vi "MOVIE_setup_acquisition_sCMOS.vi"(5 "Exposure time":dbl, 6 "Movie number":i32, 7 "Handle in":u32, 8 "error in":errorcluster, 9 "Movie folder name":string, 10 "Acquiring":bool, 11 "frames":i32) -> (0 "error out":errorcluster, 3 "t0":dbl)   [LabVIEW 2015]
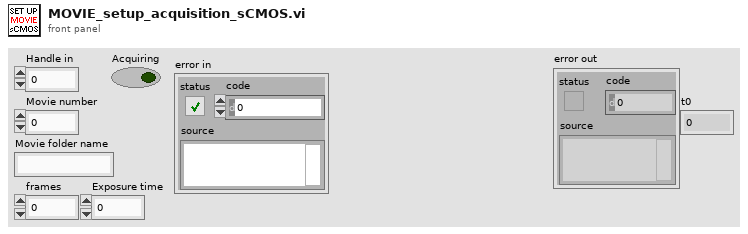
[diagram p1: front panel]
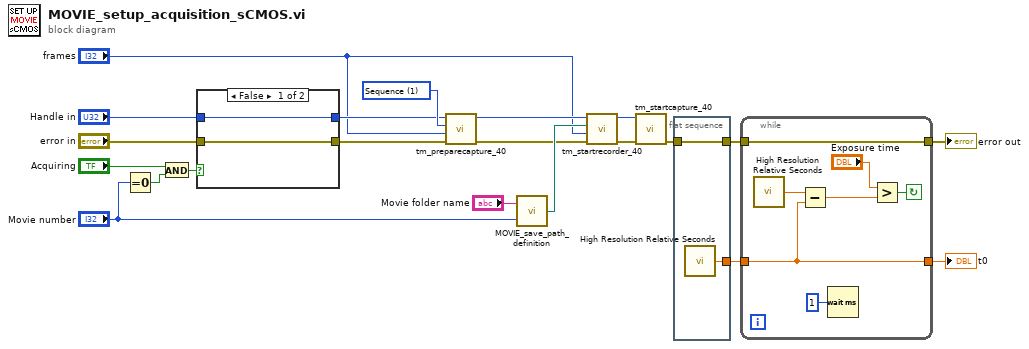
[diagram p0: block diagram]
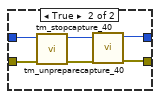
[diagram p2: hidden frame]
diagram:
  w19 = 1 items=["Snap", "Sequence"] ("Capture mode")
  n1 = Equal To 0?(x="Movie number") -> (x = 0?=w4:bool)
  n2 = And(x="Acquiring", y=w4) -> (x .and. y?=w2:bool)
  n3 = case shown="False" w2 {
    tunnel: [w23 w25] -> w14
    tunnel: "error in" -> [w23 w29]
    tunnel: "Handle in" -> [w22 w28]
    tunnel: [w22 w24] -> w15
    frame False {
    }
    frame True {
      n4 = call <userlib>:"tm_stopcapture_40.vi"("error in (no error)"=w29, "Handle in"=w28) -> ("error out"=w27:errorcluster, "Handle out"=w26:u32)  [unwired: 8 in]
      n5 = call <userlib>:"tm_unpreparecapture_40.vi"("error in (no error)"=w27, "Handle in"=w26) -> ("error out"=w25:errorcluster, "Handle out"=w24:u32)  [unwired: 8 in]
    }
  }
  n6 = call <userlib>:"tm_preparecapture_40.vi"("error in (no error)"=w14, "Frames"="frames", "Capture mode"=w19, "Handle in"=w15) -> ("error out"=w11:errorcluster, "Handle out"=w18:u32)  [unwired: 4 in, 2 out]
  n7 = call "MOVIE_save_path_definition.vi"("Movie number"="Movie number", "Movie folder name"="Movie folder name") -> ("Movie path"=w17:path)
  n8 = call <userlib>:"tm_startrecorder_40.vi"("error in (no error)"=w11, "frames"="frames", "File"=w17, "Handle in"=w18) -> ("error out"=w13:errorcluster, "Handle out"=w16:u32)  [unwired: 6 in]
  n9 = call <userlib>:"tm_startcapture_40.vi"("error in (no error)"=w13, "Handle in"=w16) -> ("error out"=w12:errorcluster)  [unwired: 8 in, 1 out]
  n10 = flat-sequence {
    tunnel: w12 -> [w31]
    tunnel: [w31] -> w7
    tunnel: [w30] -> w9
    frame #0 {
      n11 = call <vilib>:"High Resolution Relative Seconds.vi"() -> ("relative seconds"=w30:dbl)
    }
  }
  n12 = while {
    tunnel: w9 -> [w37]
    tunnel: [w37] -> w8
    tunnel: [w36] -> w6
    tunnel: w7 -> [w36]
    stop <- w33 continue-if-true
    n13 = call <vilib>:"High Resolution Relative Seconds.vi"() -> ("relative seconds"=w38:dbl)
    n14 = Subtract(x=w38, y=w37) -> (x-y=w34:dbl)
    n15 = Wait (ms)(milliseconds to wait=u32 1) -> ()  [unwired: 1 out]
    n16 = Greater?(x="Exposure time", y=w34) -> (0:w33:bool)
  }
  "error out" <- w6
  "t0" <- w8
